vi "geometry.vi"() -> ()   [LabVIEW 2013]
panel:
  out "y limit":dbl format="%#_13g"
  out "y center":dbl format="%#_13g"
  out "x limit":dbl format="%#_13g"
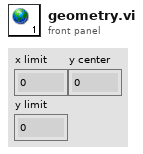
[diagram p1: front panel]
diagram:
